vi "mqttTCPIPserver.vi"(0 "mqtt in":refnum<class "mqtt.lvclass">, 11 "error in (no error)":errorcluster) -> (4 "mqtt out":refnum<class "mqtt.lvclass">, 15 "error out":errorcluster)   [LabVIEW 2017, in "mqtt.lvclass"]
uses:
  mqtt.lvclass
  mqttTXqueue/mqttTXdataQueueFunction.ctl
  mqtt.lvclass/mqtt.ctl
  mqttTypedef/mqttRXdataCluster.ctl
  mqttTypedef/mqttFixedHeaderResponse.ctl
  mqttTypedef/mqttQOSlevel.ctl
  mqttTypedef/mqttMessageType.ctl
  mqttTXqueue/mqttRXsubscriptionEventFunction.ctl
  mqttTXqueue/mqttRXsubscriptionEventData.ctl
panel:
  out "telegram":u8[](array[numeric])
  out "rxCount":i32
  out "rxTelegram":u8[](array[numeric]) format="%02x"
  out "txError":errorcluster
  out "txTelegram":u8[](array[numeric]) format="%02x"
  out "payloadError":errorcluster
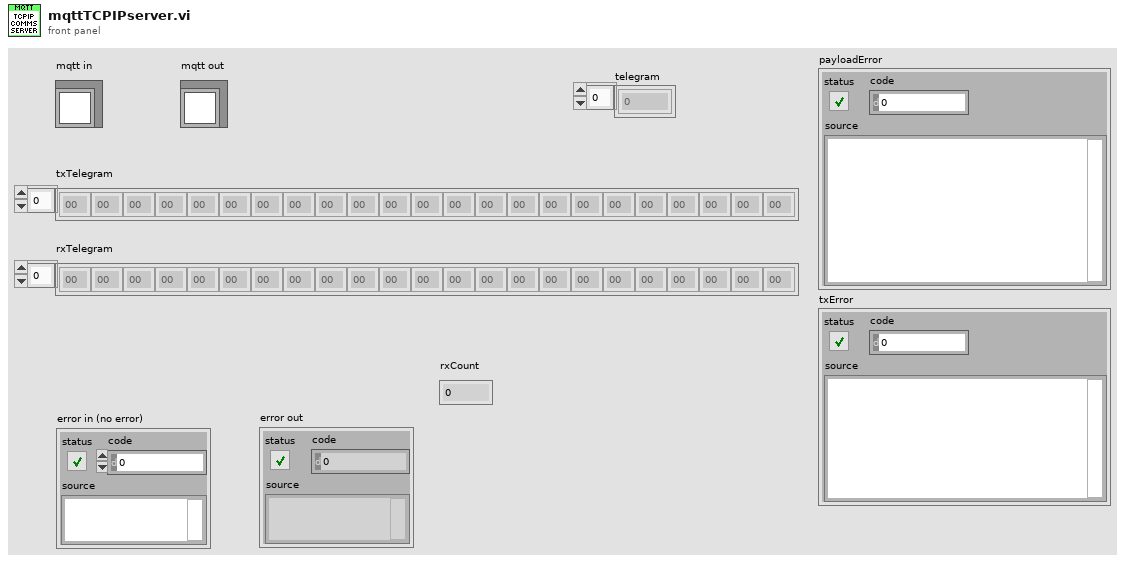
[diagram p1: front panel]
types:
  T1 = typedef "mqttTXdataQueueFunction.ctl" = enum16{"init", "deinit", "getQueue", "enqueue"}
  T2 = typedef "mqttRXdataCluster.ctl" = cluster{"fixedHdr":T3, "payload":u8[]}
  T3 = typedef "mqttFixedHeaderResponse.ctl" = cluster{"retain":bool, "qos":T4, "duplicate":bool, "response":T5}
  T4 = typedef "mqttQOSlevel.ctl" = enum8{"At most once", "At least once", "Exactly once", "Reserved"}
  T5 = typedef "mqttMessageType.ctl" = enum32{"Reserved", "CONNECT", "CONNACK", "PUBLISH", "PUBACK", "PUBREC", "PUBREL", "PUBCOMP", "SUBSCRIBE", "SUBACK", "UNSUBSCRIBE", "UNSUBACK", "PINGREQ", "PINGRESP", "DISCONNECT", "Reserved2"}
  T6 = typedef "mqttRXsubscriptionEventData.ctl" = cluster{"topic":string, "value":string, "messageID":u16}
  T7 = typedef "mqttRXsubscriptionEventFunction.ctl" = enum16{"init", "deinit", "getEventRef", "event"}
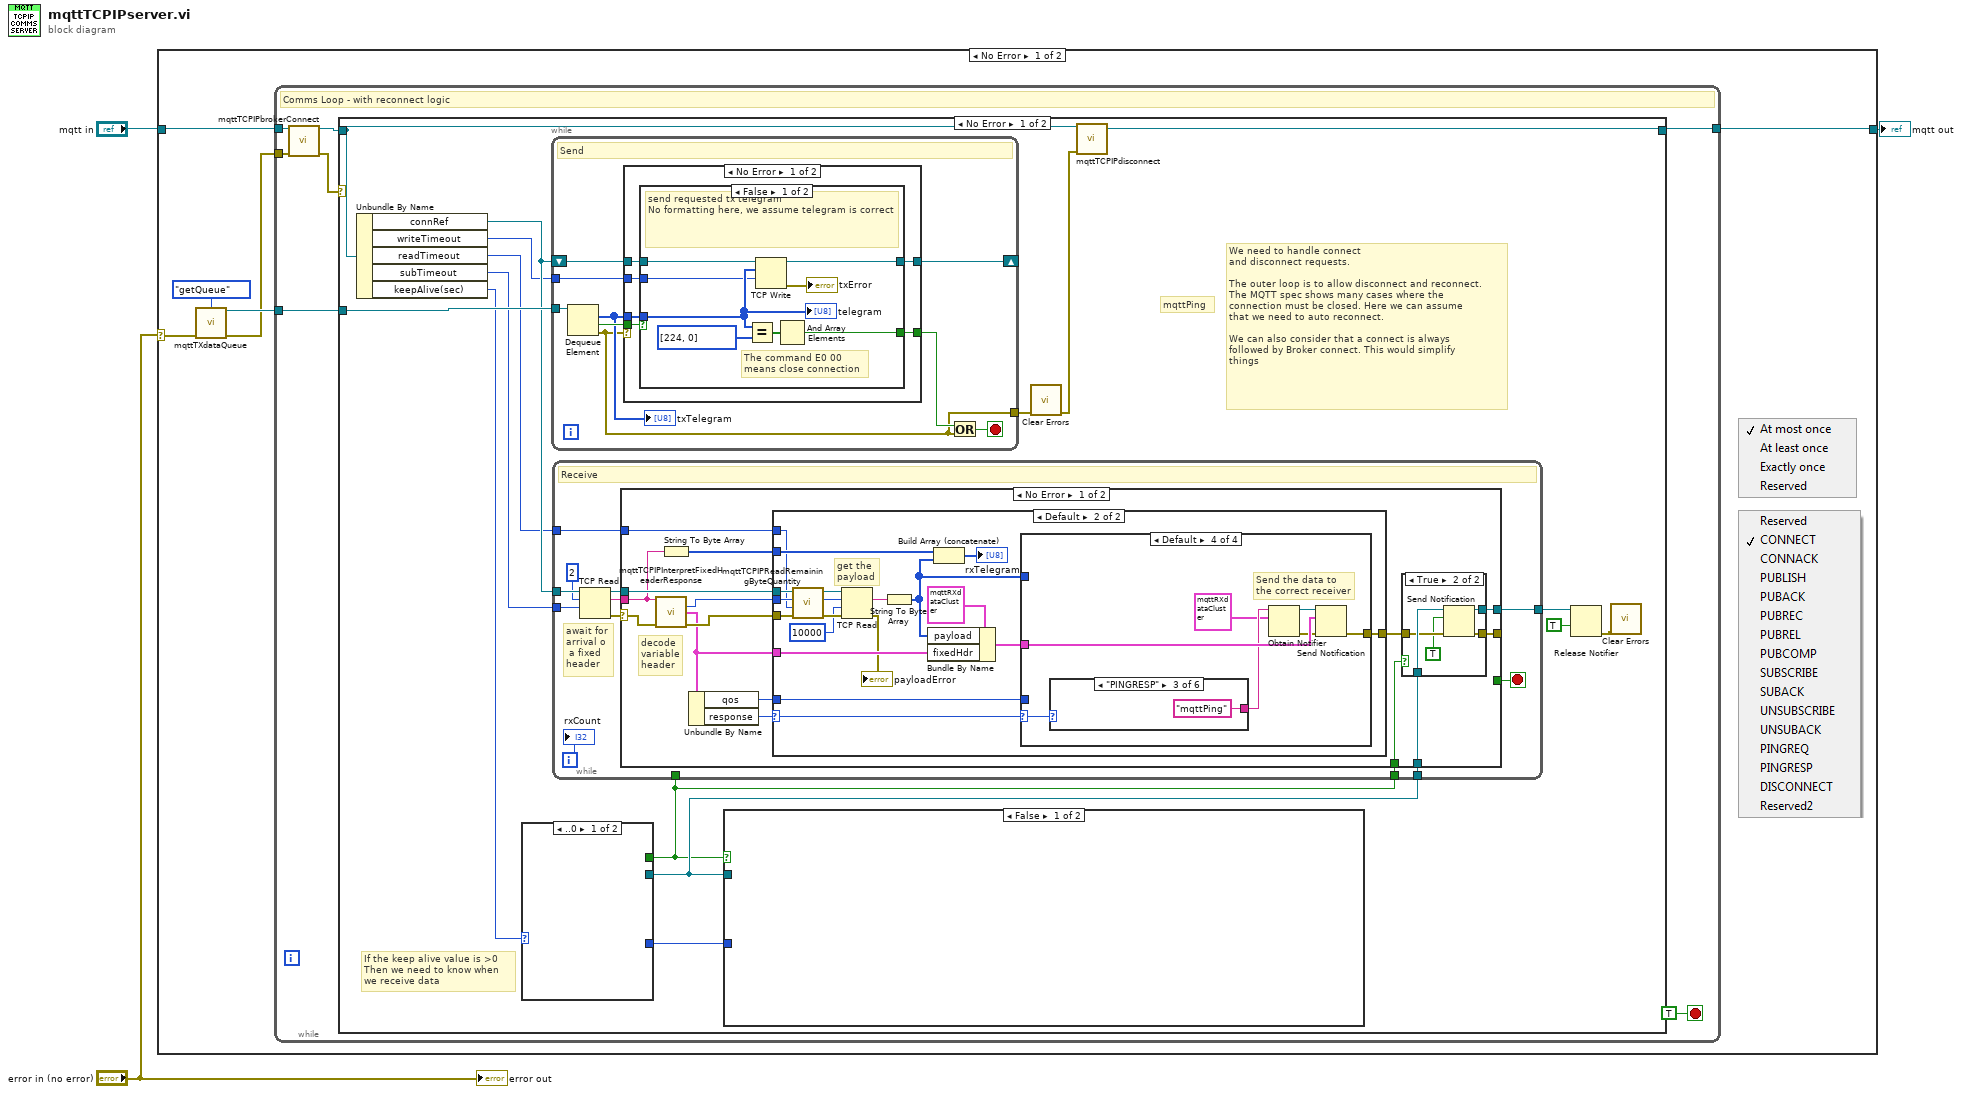
[diagram p0: block diagram]
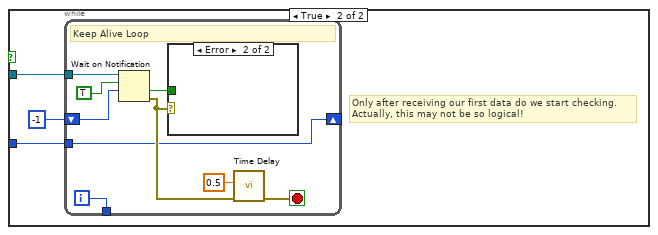
[diagram p2: hidden frame]
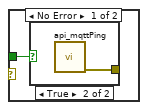
[diagram p3: hidden frame]
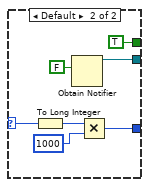
[diagram p5: hidden frame]
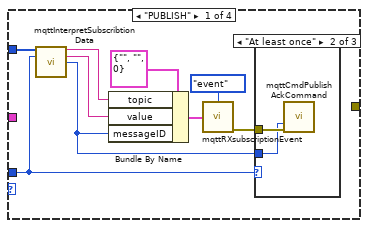
[diagram p8: hidden frame]
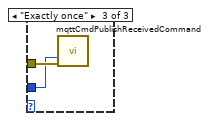
[diagram p10: hidden frame]
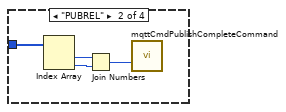
[diagram p11: hidden frame]
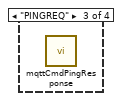
[diagram p12: hidden frame]
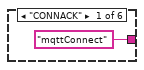
[diagram p13: hidden frame]
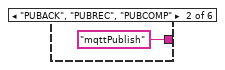
[diagram p14: hidden frame]
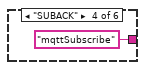
[diagram p15: hidden frame]
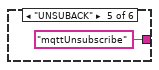
[diagram p16: hidden frame]
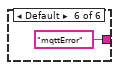
[diagram p17: hidden frame]
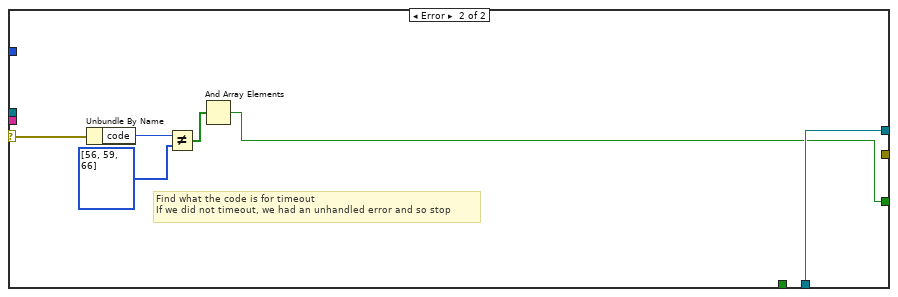
[diagram p18: hidden frame]
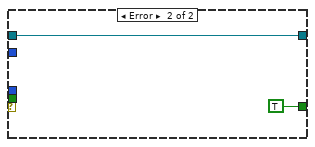
[diagram p20: hidden frame]
diagram:
  n1 = case shown="No Error" "error in (no error)" {
    selector: "error in (no error)" -> [w4 _]
    tunnel: "mqtt in" -> [w7 w172]
    tunnel: [w6 w172] -> w2
    frame No Error {
      n2 = call "mqttTXdataQueue.vi"("function"=mqttTXdataQueueFunction."getQueue", "error in (no error)"=w4) -> ("Queue out"=w9:refnum<queue>, "error out"=w5:errorcluster)  [unwired: 12 in]
      n3 = while {
        tunnel: w9 -> [w16]
        tunnel: w7 -> [w14]
        tunnel: [w12] -> w6
        tunnel: w5 -> [w13]
        stop <- TRUE stop-if-true
        # "Comms Loop - with reconnect logic"
        n4 = call "mqttTCPIPbrokerConnect.vi"("mqtt in"=w14, "error in (no error)"=w13) -> ("mqtt out"=w11:refnum<class "mqtt.lvclass">, "error out"=w10:errorcluster)  [unwired: 12 in]
        n5 = case shown="No Error" w10 {
          selector: w10 -> [_ w168]
          tunnel: w16 -> [w32 _]
          tunnel: [w28 w171] -> w12
          tunnel: w11 -> [w27 w171]
          frame No Error {
            # "If the keep alive value is >0\nThen we need to know when\nwe receive data"
            # "mqttPing"
            # "We need to handle connect\nand disconnect requests.\n\nThe outer loop is to allow disconnect and reconnect.\nThe MQTT spec shows many cases where the\nconnection must be closed. Here we can assume\nthat we need to auto reconnect.\n\nWe can also consider that a connect is always\nfollowed by Broker connect. This would simplify\nthings"
            n6 = Unbundle By Name(w27) -> ("connRef"=w31:refnum<k5>, "writeTimeout"=w26:i32, "readTimeout"=w25:i32, "subTimeout"=w24:i32, "keepAlive(sec)"=w18:u16)
            n7 = case shown="..0" w18 {
              selector: w18 -> [_ w48]
              tunnel: [_ w53] -> w23
              tunnel: [_ w49] -> w19
              tunnel: [_ TRUE] -> w17
              frame ..0 {
              }
              frame Default {
                n8 = To Long Integer(number=w48) -> (32bit integer=w51:i32)
                n9 = Obtain Notifier(notification data type=FALSE) -> (notifier out=w53:refnum<notifier>)  [unwired: 3 in, 2 out]
                n10 = Multiply(x=w51, y=1000) -> (x*y=w49:i32)
              }
            }
            n11 = while {
              tunnel: w32 -> [w149]
              shift-right: [w146] -> _
              shift-left: w31 -> [w147]
              tunnel: [w142] -> w30
              tunnel: w26 -> [w141]
              stop <- w145 stop-if-true
              # "Send"
              n12 = Dequeue Element(queue=w149) -> (element=w143:u8[], timed out?=w148:bool, error out=w142:errorcluster)  [unwired: 2 in, 1 out]
              "txTelegram" <- w143
              n13 = case shown="No Error" w142 {
                tunnel: w148 -> [w155 _]
                tunnel: w143 -> [w154 _]
                tunnel: w147 -> [w153 w166]
                tunnel: [w152 w166] -> w146
                tunnel: [w151 TRUE] -> w144
                tunnel: w141 -> [w150 _]
                frame No Error {
                  n14 = case shown="False" w155 {
                    tunnel: w154 -> [w161 _]
                    tunnel: w153 -> [w163 w164]
                    tunnel: [w162 w164] -> w152
                    tunnel: [w158 _] -> w151
                    tunnel: w150 -> [w156 _]
                    frame False {
                      # "The command E0 00\nmeans close connection"
                      # "send requested tx telegram\nNo formatting here, we assume telegram is correct"
                      n15 = Equal?(x=w161, y=u8[] [224, 0] ("txTelegram 2")) -> (x = y?=w159:bool[])
                      n16 = TCP Write(connection ID=w163, data in=w161, 9:w156) -> (connection ID out=w162:refnum<k5>, error out=→"txError":errorcluster)  [unwired: 1 in, 1 out]
                      n17 = And Array Elements(Boolean array=w159) -> (logical AND=w158:bool)
                      "telegram" <- w161
                    }
                    frame True {
                      # "Queue Timed Out - do nothing.\nWe can later use this for the Keep Alive ping"
                    }
                  }
                }
                frame Error {
                }
              }
              n18 = Or(x=w144, y=w142) -> (x .or. y?=w145:bool)
            }
            n19 = while {
              tunnel: w31 -> [w65]
              tunnel: w25 -> [w59]
              tunnel: w24 -> [w58]
              tunnel: w23 -> [w57]
              tunnel: [w56] -> w22
              tunnel: w17 -> [w55]
              tunnel: w17 -> [_]
              i -> [w60]
              stop <- w61 stop-if-true
              # "await for\narrival o\n a fixed\nheader"
              # "Receive"
              n20 = TCP Read(connection ID=w65, bytes to read=2, 9:w58) -> (connection ID out=w64:refnum<k5>, data out=w62:string, error out=w54:errorcluster)  [unwired: 2 in]
              n21 = case shown="No Error" w54 {
                selector: w54 -> [w78 w140]
                tunnel: w64 -> [w79 _]
                tunnel: w62 -> [w74 _]
                tunnel: [_ w135] -> w61
                tunnel: w59 -> [w71 _]
                tunnel: w57 -> [w70 w137]
                tunnel: [w68 w137] -> w56
                tunnel: [w67 _] -> _
                tunnel: w55 -> [w66 _]
                frame No Error {
                  # "decode\nvariable\nheader"
                  n22 = call "mqttTCPIPInterpretFixedHeaderResponse.vi"("data in"=w74, "error in (no error)"=w78) -> ("remainingLengthByte1"=w80:u8, "output cluster"=w76:T3, "error out"=w77:errorcluster)  [unwired: 11 in]
                  n23 = String To Byte Array(string=w74) -> (unsigned byte array=w73:u8[])
                  n24 = Unbundle By Name(w76) -> ("qos"=w72:T4, "response"=w75:T5)
                  n25 = case shown="Default" w75 {
                    selector: w75 -> [_ w94]
                    tunnel: w80 -> [_ w104]
                    tunnel: w79 -> [_ w103]
                    tunnel: w77 -> [_ w96]
                    tunnel: w76 -> [_ w95]
                    tunnel: w73 -> [_ w91]
                    tunnel: w72 -> [_ w90]
                    tunnel: w71 -> [_ w87]
                    tunnel: [_ w86] -> w69
                    frame "CONNECT", "SUBSCRIBE" {
                      # "The client should not receive these commands.\nI had some problems with these commands being received\nand it appears this was a broker issue. However, to ignore\nmessages that we should not receive is no bad thing."
                    }
                    frame Default {
                      # "get the\npayload"
                      n26 = call "mqttTCPIPReadRemainingByteQuantity.vi"("error in (no error)"=w96, "readTimeout ms (2000)"=w87, "remainingLengthByte1"=w104, "connRef in"=w103) -> ("error out"=w101:errorcluster, "remainingLength"=w100:i32, "connRef out"=w102:refnum<k5>)  [unwired: 5 in]
                      n27 = TCP Read(connection ID=w102, bytes to read=w100, error in (no error)=w101, 9:10000 ("timeout ms (25000)")) -> (data out=w98:string, error out=→"payloadError":errorcluster)  [unwired: 1 in, 1 out]
                      n28 = String To Byte Array(string=w98) -> (unsigned byte array=w88:u8[])
                      n29 = Bundle By Name(cluster=T2 {"fixedHdr"={"retain"=FALSE, "qos"=enum."At most once", "duplicate"=FALSE, "response"=enum."Reserved"}, "payload"=[]} ("output cluster"), "payload"=w88, "fixedHdr"=w95) -> (w92:T2)
                      n30 = Build Array (concatenate)(w91, w88) -> (→"rxTelegram":u8[])
                      n31 = case shown="Default" w94 {
                        selector: w94 -> [_ _ _ w128]
                        tunnel: w92 -> [_ _ _ w127]
                        tunnel: w90 -> [w106 _ _ _]
                        tunnel: w88 -> [w110 w121 _ _]
                        tunnel: [_ _ _ w122] -> w86
                        frame "PUBLISH" {
                          n32 = call "mqttInterpretSubscribtionData.vi"("rxTelegram in"=w110, "qos"=w106) -> ("topic"=w109:string, "value"=w108:string, "messageID"=w105:u16)  [unwired: 10 in, 1 out]
                          n33 = Bundle By Name(cluster=T6 {"topic"="", "value"="", "messageID"=0} ("data"), "topic"=w109, "value"=w108, "messageID"=w105) -> (w111:T6)
                          n34 = call "mqttRXsubscriptionEvent.vi"("function"=mqttRXsubscriptionEventFunction."event", "data"=w111) -> ("error out"=w107:errorcluster)  [unwired: 12 in, 1 out]
                          n35 = case shown="\"At least once\"" w106 {
                            tunnel: w107 -> [_ w115 w117]
                            tunnel: w105 -> [_ w114 w116]
                            frame Default {
                            }
                            frame "At least once" {
                              n36 = call "mqttCmdPublishAckCommand.vi"("messageID"=w114, "error in (no error)"=w115) -> ()  [unwired: 13 in, 1 out]
                            }
                            frame "Exactly once" {
                              n37 = call "mqttCmdPublishReceivedCommand.vi"("messageID"=w116, "error in (no error)"=w117) -> ()  [unwired: 13 in, 1 out]
                            }
                          }
                        }
                        frame "PUBREL" {
                          n38 = Index Array(array=w121) -> (element #1=w120:u8, element #2=w119:u8)  [unwired: 2 in]
                          n39 = Join Numbers(hi=w120, lo=w119) -> ((hi.lo)=w118:u16)
                          n40 = call "mqttCmdPublishCompleteCommand.vi"("messageID"=w118) -> ()  [unwired: 14 in, 1 out]
                        }
                        frame "PINGREQ" {
                          n41 = call "mqttCmdPingResponse.vi"() -> ()  [unwired: 15 in, 1 out]
                        }
                        frame Default {
                          # "Send the data to\nthe correct receiver"
                          n42 = case shown="\"PINGRESP\"" w128 {
                            tunnel: ["mqttConnect" ("name (unnamed)") "mqttPublish" ("name (unnamed)") "mqttPing" ("name (unnamed)") "mqttSubscribe" ("name (unnamed)") "mqttUnsubscribe" ("name (unnamed)") "mqttError" ("name (unnamed)")] -> w126
                            frame "CONNACK" {
                            }
                            frame "PUBACK", "PUBREC", "PUBCOMP" {
                            }
                            frame "PINGRESP" {
                            }
                            frame "SUBACK" {
                            }
                            frame "UNSUBACK" {
                            }
                            frame Default {
                            }
                          }
                          n43 = Obtain Notifier(name (unnamed)=w126, notification data type=T2 {"fixedHdr"={"retain"=FALSE, "qos"=enum."At most once", "duplicate"=FALSE, "response"=enum."Reserved"}, "payload"=[]} ("output cluster")) -> (notifier out=w125:refnum<notifier>, error out=w123:errorcluster)  [unwired: 2 in, 1 out]
                          n44 = Send Notification(notification=w127, notifier=w125, error in (no error)=w123) -> (error out=w122:errorcluster)  [unwired: 1 out]
                        }
                      }
                    }
                  }
                  n45 = case shown="True" w66 {
                    tunnel: w70 -> [_ w85]
                    tunnel: w69 -> [_ w84]
                    tunnel: [_ w82] -> w68
                    tunnel: [_ w81] -> w67
                    frame False {
                    }
                    frame True {
                      n46 = Send Notification(notification=TRUE, notifier=w85, error in (no error)=w84) -> (notifier out=w82:refnum<notifier>, error out=w81:errorcluster)
                    }
                  }
                }
                frame Error {
                  # "Find what the code is for timeout\nIf we did not timeout, we had an unhandled error and so stop"
                  n47 = Unbundle By Name(w140) -> ("code"=w139:i32)
                  n48 = Not Equal?(x=w139, y=i32[] [56, 59, 66]) -> (x != y?=w136:bool[])
                  n49 = And Array Elements(Boolean array=w136) -> (logical AND=w135:bool)
                }
              }
              "rxCount" <- w60
            }
            n50 = case shown="False" w17 {
              tunnel: w23 -> [_ w35]
              tunnel: w19 -> [_ w34]
              frame False {
              }
              frame True {
                # "Only after receiving our first data do we start checking.\nActually, this may not be so logical!"
                n51 = while {
                  tunnel: w35 -> [w44]
                  tunnel: [w39] -> _
                  shift-right: [w36] -> _
                  shift-left: -1 -> [w43]
                  tunnel: w34 -> [w36]
                  i -> [w39]
                  stop <- w40 stop-if-true
                  # "Keep Alive Loop"
                  n52 = Wait on Notification(notifier=w44, ignore previous (F)=TRUE, timeout in ms (-1)=w43) -> (timed out?=w42:bool, error out=w37:errorcluster)  [unwired: 1 in, 2 out]
                  n53 = case shown="Error" w37 {
                    tunnel: w42 -> [w45 _]
                    frame No Error {
                      n54 = case shown="True" w45 {
                        tunnel: [_ w46] -> _
                        frame False {
                        }
                        frame True {
                          n55 = call "api_mqttPing.vi"() -> ("error out"=w46:errorcluster)  [unwired: 14 in, 1 out]
                        }
                      }
                    }
                    frame Error {
                    }
                  }
                  n56 = call "Time Delay"("error in (no error)"=w37, "Delay Time (s)"=0.5) -> ("error out"=w40:errorcluster)  [unwired: 9 in]
                }
              }
            }
            n57 = call <vilib>:"Clear Errors.vi"("error in (no error)"=w30) -> ("error out"=w29:errorcluster)  [unwired: 5 in, 1 out]
            n58 = call "mqttTCPIPdisconnect.vi"("mqtt in"=w27, "error in (no error)"=w29) -> ("mqtt out"=w28:refnum<class "mqtt.lvclass">)  [unwired: 12 in, 1 out]
            n59 = Release Notifier(notifier=w22, force destroy? (F)=TRUE) -> (error out=w20:errorcluster)  [unwired: 1 in, 2 out]
            n60 = call <vilib>:"Clear Errors.vi"("error in (no error)"=w20) -> ()  [unwired: 5 in, 2 out]
          }
          frame Error {
            w167 = T2 {"fixedHdr"={"retain"=FALSE, "qos"=enum."At most once", "duplicate"=FALSE, "response"=enum."Reserved"}, "payload"=[]} ("output cluster")
            n61 = Obtain Notifier(notification data type=w167, error in (no error)=w168) -> (notifier out=w170:refnum<notifier>, error out=w169:errorcluster)  [unwired: 2 in, 1 out]
            n62 = Send Notification(notification=w167, notifier=w170, error in (no error)=w169) -> ()  [unwired: 2 out]
          }
        }
      }
    }
    frame Error {
    }
  }
  "mqtt out" <- w2
  "error out" <- "error in (no error)"
